vi "Initialize Attributes.vi"(8 "error in (no error)":errorcluster, 10 "Attribute Data":variant, 11 "CS++Scope":refnum<class "CS++Scope.lvclass">) -> (0 "error out":errorcluster, 2 "Found?":bool, 3 "CS++Scope out":refnum<class "CS++Scope.lvclass">)   [LabVIEW 2014, in "CS++Scope.lvlib" / "CS++Scope.lvclass"]
doc: "Initialize object attribute.\n\nUnique resources should be allocated elsewhere!"
uses:
  CS++Scope.lvclass
  PV-Enum.ctl
  PV-Enum-n.ctl
  CSPP_Core/Classes/CS++ProcessVariables/ProcessVariable/PV.lvclass
  CSPP_Core/Classes/CS++ProcessVariables/ProcessVariable/PV.lvclass/PV.ctl
  CSPP_Core/Actors/CS++BaseActor/CS++BaseActor.lvclass/CS++BaseActor.ctl
  CS++Scope.lvclass/CS++Scope.ctl
  CSPP_Core/Classes/CS++ProcessVariables/ProcessVariable/Write PV URL.vi
  CSPP_Core/Classes/CS++ProcessVariables/ProcessVariable/Write Type Descriptor.vi
  CSPP_Core/Actors/CS++DeviceActor/CS++DeviceActor.lvclass
  CSPP_Core/Classes/CS++BaseClasses/Factory/CS++Factory.lvclass
  CSPP_Core/Actors/CS++BaseActor/CS++BaseActor.lvclass
  CSPP_Core/Libraries/Utilities/CS++Utilities.lvlib
  CSPP_Core/Classes/CS++ProcessVariables/CS++ProcessVariables.lvlib
panel:
  in  "PV-Enum-n":T1
  in  "PV-Enum":T2
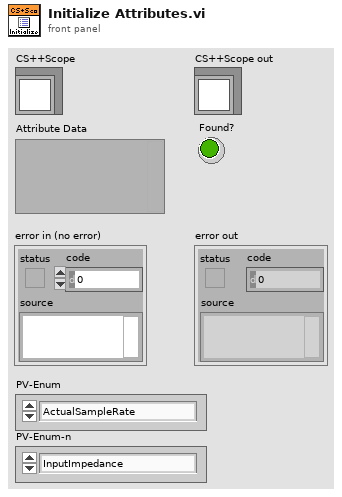
[diagram p1: front panel]
types:
  T1 = typedef "CS++Scope.lvlib/CS++Scope.lvclass/PV-Enum-n.ctl" = enum16{"InputImpedance", "MaxInputFrequency", "VerticalRange", "ProbeAttenuation", "VerticalOffset", "VerticalCoupling", "ChannelEnabled"}
  T2 = typedef "CS++Scope.lvlib/CS++Scope.lvclass/PV-Enum.ctl" = enum16{"ActualSampleRate", "TimePerRecord", "AcquisitionStartTime", "TriggerLevel", "GlitchWidth", "LowReference", "MidReference", "HighReference", "RuntLowThreshold", "RuntHighThreshold", "TriggerHoldoff", "WidthLowThreshold", "WidthHighThreshold", "AcquisitionStatus", "ActualRecordLength", "ActualSampleMode", "ACLineTriggerSlope", "MinRecordLength", "AcquisitionType", "TriggerSlope", "GlitchCondition", "GlitchPolarity", "InterpolationMethod", "NumberOfAverages", "NumberOfEnvelopes", "TriggerType", "TriggerCoupling", "TriggerModifier", "TVLineNumber", "TVEvent", "TVTriggerPolarity", "TVSignalFormat", "WidthCondition", "WidthPolarity", "MeasurementDone", "ContinousAcquisition", "TriggerSource", "Waveform", "ActualTimeIncrement"}
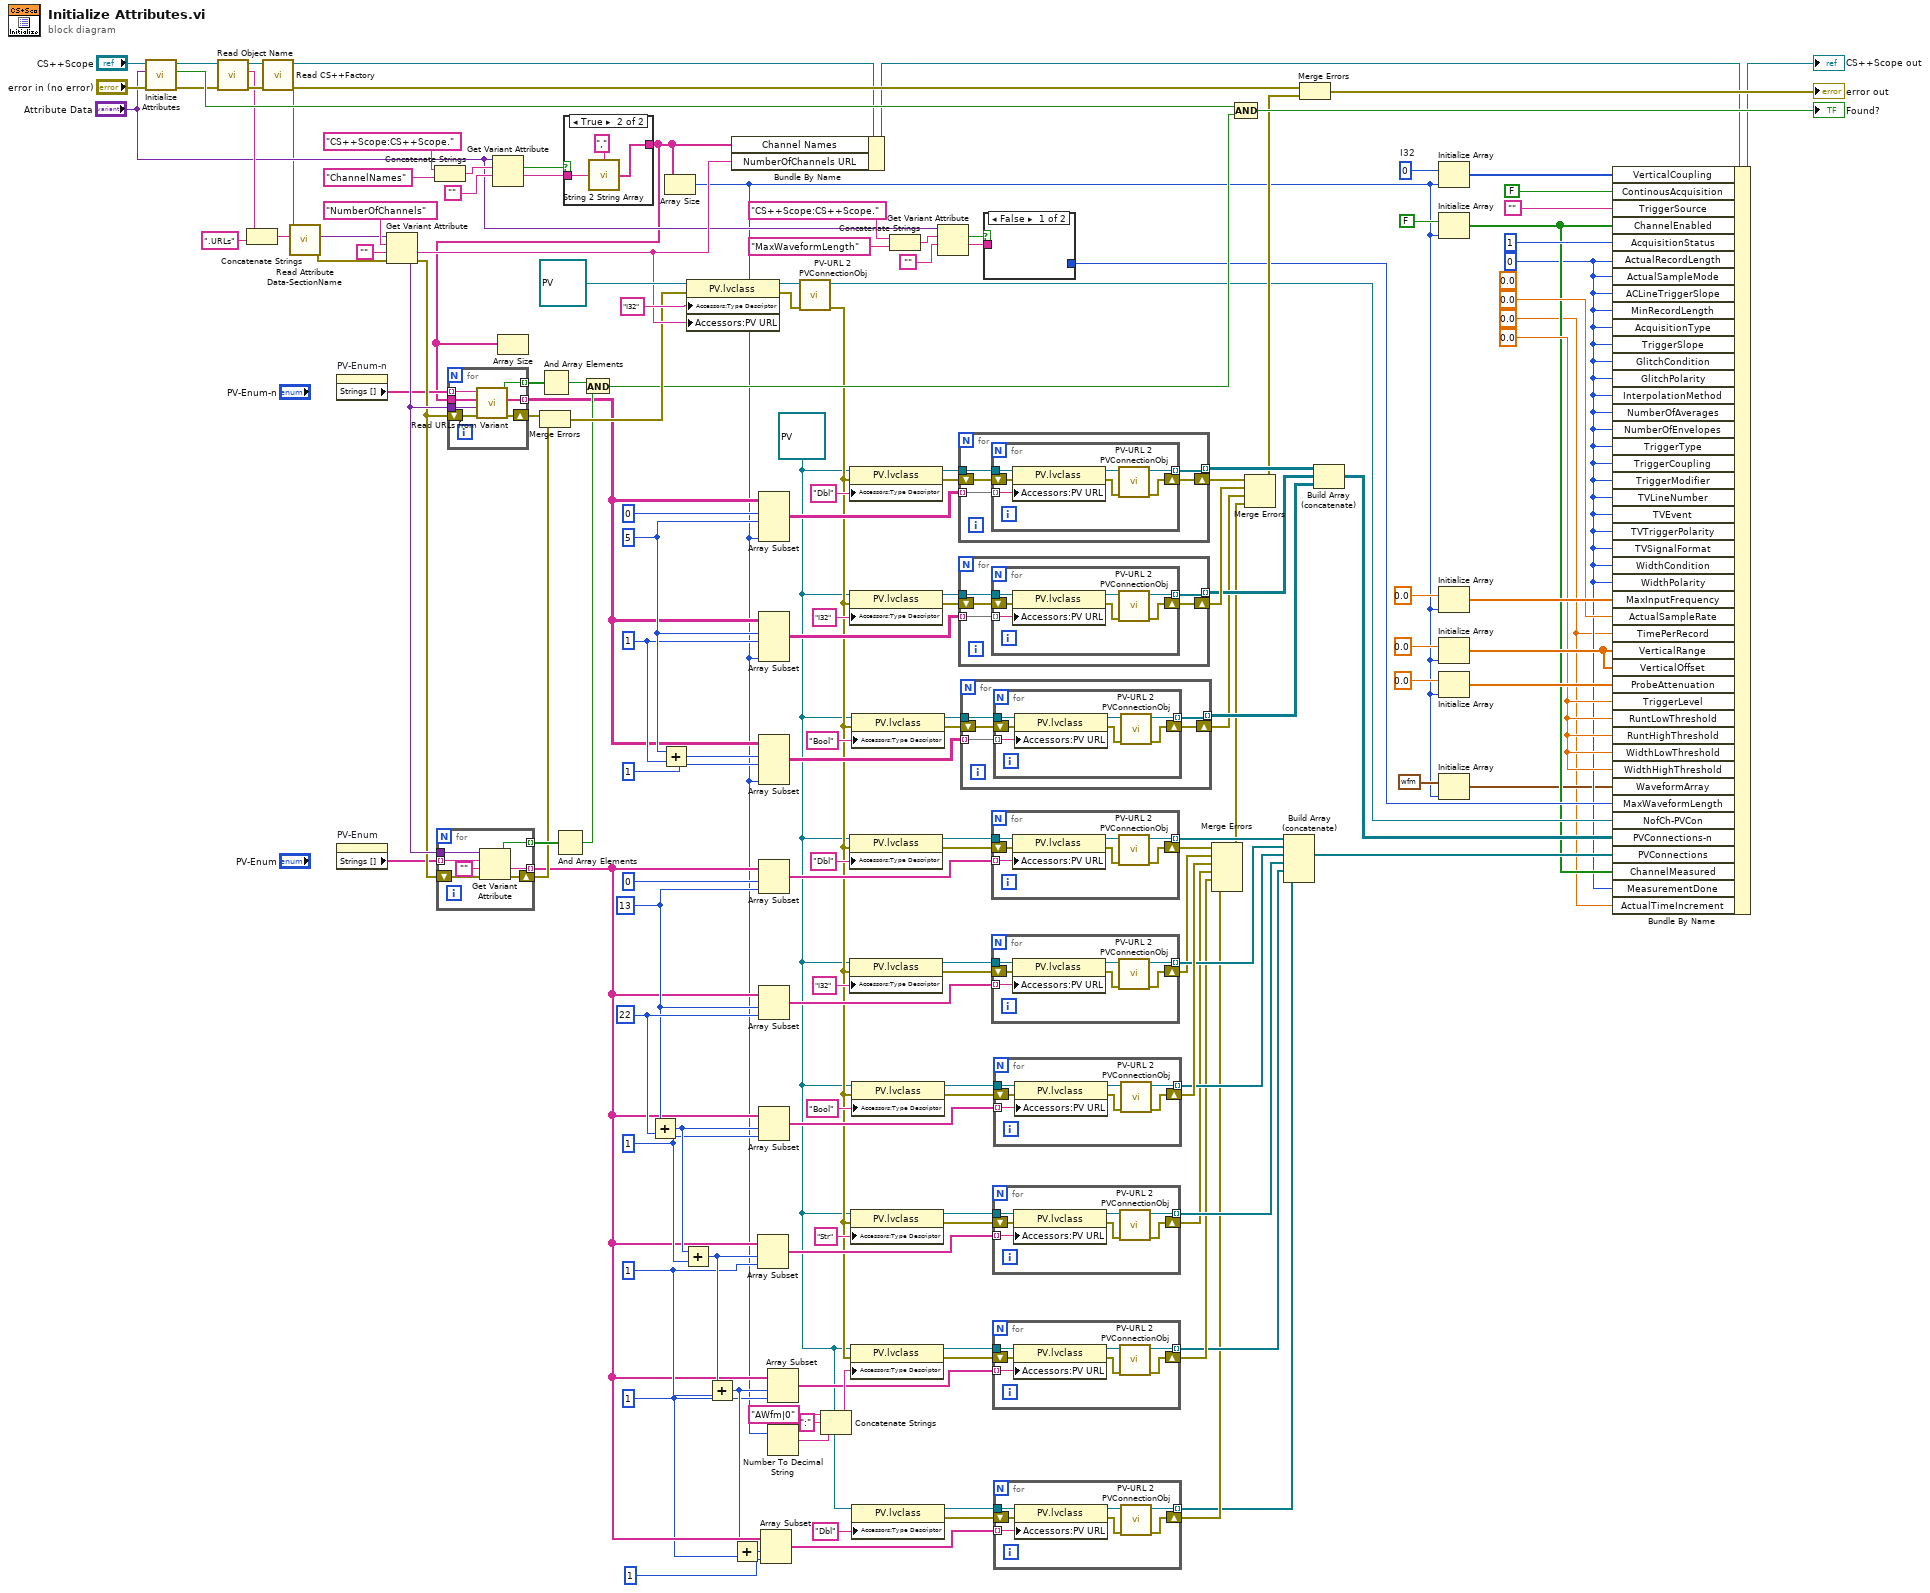
[diagram p0: block diagram]
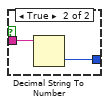
[diagram p2: hidden frame]
diagram:
  w7 = 1 ("length")
  w50 = dbl[unit] 0.0 ("modulation depth (0.00 %)")
  w19 = dbl[unit] 0.0 ("modulation depth (0.00 %)")
  w21 = 1 ("length")
  w58 = 1 ("length")
  w96 = 22 ("length")
  w95 = 13 ("length")
  w103 = 1 ("length")
  w104 = 5 ("length")
  w13 = refnum<class "PV.lvclass"> refnum ("CS++ProcessVariables.lvlib:PV.lvclass")
  (unwired) 0.0 ("modulation depth (0.00 %)")
  w35 = 0 ("I32")
  w136 = 0  # I32
  n1 = call-parent "Initialize Attributes.vi"("error in (no error)"="error in (no error)", "Attribute Data"="Attribute Data", "CS++DeviceActor in"="CS++Scope") -> ("error out"=w151:errorcluster, "Found?"=w154:bool, "CS++DeviceActor out"=w130:refnum<class "CS++Scope.lvclass">)  [unwired: 6 in]
  n2 = call "Read Object Name.vi"("error in (no error)"=w151, "CS++BaseActor in"=w130) -> ("error out"=w152:errorcluster, "Object Name"=w138:string, "CS++BaseActor out"=w153:refnum<class "CS++Scope.lvclass">)  [unwired: 7 in]
  n3 = Concatenate Strings(w138, ".URLs" ("string")) -> (w4:string)
  n4 = call "Read CS++Factory.vi"("error in (no error)"=w152, "CS++BaseActor in"=w153) -> ("error out"=w150:errorcluster, "CS++Factory"=w3:refnum<class "CS++Factory.lvclass">, "CS++BaseActor out"=w143:refnum<class "CS++Scope.lvclass">)  [unwired: 7 in]
  n5 = call-dynamic "Read Attribute Data-SectionName.vi"("Object Name"=w4, "CS++Factory in"=w3) -> ("error out"=w6:errorcluster, "Attribute Data"=w5:variant)  [unwired: 7 in, 1 out]
  n6 = property on="PV-Enum-n" class="Enum (strict)"() -> ("Strings []"=w66:string[])  [unwired: 2 in, 2 out]
  n7 = property on="PV-Enum" class="Enum (strict)"() -> ("Strings []"=w65:string[])  [unwired: 2 in, 2 out]
  n8 = Get Variant Attribute(Variant=w5, name="NumberOfChannels" ("string"), default value (empty Variant)="", error in=w6) -> (duplicate Variant=w101:variant, value=w125:string, error out=w100:errorcluster)  [unwired: 1 out]
  n9 = Concatenate Strings("CS++Scope:CS++Scope.", "ChannelNames" ("string")) -> (w145:string)
  n10 = for {
    tunnel: w65 -> [w159] mode=indexing
    tunnel: w101 -> [w160]
    shift-right: [w162] -> w73
    shift-left: w100 -> [w161]
    tunnel: [w158] -> w75 mode=indexing
    tunnel: [w156] -> w12 mode=indexing
    n11 = Get Variant Attribute(Variant=w160, name=w159, default value (empty Variant)="", error in=w161) -> (found=w158:bool, value=w156:string, error out=w162:errorcluster)  [unwired: 1 out]
  }
  n12 = Get Variant Attribute(Variant="Attribute Data", name=w145, default value (empty Variant)="") -> (found=w148:bool, value=w147:string)  [unwired: 1 in, 2 out]
  n13 = And Array Elements(Boolean array=w75) -> (logical AND=w71:bool)
  n14 = case shown="True" w148 {
    tunnel: w147 -> [_ w165]
    tunnel: [_ w164] -> w34
    frame False {
    }
    frame True {
      n15 = call "String 2 String Array.vi"("String"=w165, "Delimiter (\",\")"="," ("Delimiter (\",\")")) -> ("Substrings"=w164:string[])
    }
  }
  n16 = for {
    tunnel: w66 -> [w172] mode=indexing
    tunnel: [w171] -> w124 mode=indexing
    tunnel: w101 -> [w169]
    tunnel: w34 -> [w168]
    tunnel: [w167] -> w41 mode=indexing
    shift-right: [w170] -> w102
    shift-left: w100 -> [w166]
    n17 = call "Read URLs from Variant.vi"("Error In"=w166, "URL Section Data"=w169, "Channel Names"=w168, "URL Prefix"=w172) -> ("Error Out"=w170:errorcluster, "URLs"=w167:string[], "Found?"=w171:bool)  [unwired: 5 in]
  }
  n18 = Array Size(array=w34) -> ()  [unwired: 1 out]
  n19 = Merge Errors(w102, w73) -> (w74:errorcluster)
  n20 = And Array Elements(Boolean array=w124) -> (logical AND=w97:bool)
  n21 = And(x=w97, y=w71) -> (x .and. y?=w72:bool)
  n22 = Add(x=w95, y=w96) -> (x+y=w59:i32)
  n23 = Add(x=w104, y=w103) -> (x+y=w40:i32)
  n24 = Array Size(array=w34) -> (size(s)=w2:i32)
  n25 = Add(x=w59, y=w58) -> (x+y=w22:i32)
  n26 = property class="PV.lvclass"(reference=refnum<class "PV.lvclass"> refnum ("CS++ProcessVariables.lvlib:PV.lvclass"), error in=w74, "Accessors:Type Descriptor"="I32" ("Type Descriptor"), "Accessors:PV URL"=w125) -> (reference out=w126:refnum<class "PV.lvclass">, error out=w127:errorcluster)
  n27 = Add(x=w22, y=w21) -> (x+y=w8:i32)
  n28 = Bundle By Name(cluster=w143, "Channel Names"=w34, "NumberOfChannels URL"=w125) -> (w99:refnum<class "CS++Scope.lvclass">)
  n29 = Add(x=w8, y=w7) -> (x+y=w9:i32)
  n30 = Array Subset(array=w12, index=w22, length=w21) -> (w60:string[])
  n31 = Array Subset(array=w41, index (row)=0 ("index"), length (row)=w104, length (col)=w2) -> (w123:string[][])  [unwired: 1 in]
  n32 = Array Subset(array=w41, index (row)=w104, length (row)=w103, length (col)=w2) -> (w112:string[][])  [unwired: 1 in]
  n33 = Array Subset(array=w41, index (row)=w40, length (row)=1 ("length"), length (col)=w2) -> (w111:string[][])  [unwired: 1 in]
  n34 = Array Subset(array=w12, index=0, length=w95) -> (w76:string[])
  n35 = Array Subset(array=w12, index=w95, length=w96) -> (w87:string[])
  n36 = Array Subset(array=w12, index=w59, length=w58) -> (w88:string[])
  n37 = Array Subset(array=w12, index=w9, length=1) -> (w14:string[])
  n38 = Array Subset(array=w12, index=w8, length=w7) -> (w23:string[])
  n39 = Number To Decimal String(number=w2) -> (decimal integer string=w30:string)  [unwired: 1 in]
  n40 = call "PV-URL 2 PVConnectionObj.vi"("Error In"=w127, "PV"=w126) -> ("Error Out"=w24:errorcluster, "PVConnection"=w49:refnum<class "PVConnection.lvclass">)  [unwired: 7 in, 1 out]
  n41 = Concatenate Strings("AWfm|0" ("Type Descriptor"), ":" ("string"), w30) -> (w29:string)
  n42 = property class="PV.lvclass"(reference=w13, error in=w24, "Accessors:Type Descriptor"="Dbl" ("Type Descriptor")) -> (reference out=w121:refnum<class "PV.lvclass">, error out=w120:errorcluster)
  n43 = property class="PV.lvclass"(reference=w13, error in=w24, "Accessors:Type Descriptor"="I32" ("Type Descriptor")) -> (reference out=w116:refnum<class "PV.lvclass">, error out=w117:errorcluster)
  n44 = property class="PV.lvclass"(reference=w13, error in=w24, "Accessors:Type Descriptor"="Dbl" ("Type Descriptor")) -> (reference out=w78:refnum<class "PV.lvclass">, error out=w79:errorcluster)
  n45 = property class="PV.lvclass"(reference=w13, error in=w24, "Accessors:Type Descriptor"="I32" ("Type Descriptor")) -> (reference out=w83:refnum<class "PV.lvclass">, error out=w82:errorcluster)
  n46 = property class="PV.lvclass"(reference=w13, error in=w24, "Accessors:Type Descriptor"="Str" ("Type Descriptor")) -> (reference out=w62:refnum<class "PV.lvclass">, error out=w63:errorcluster)
  n47 = property class="PV.lvclass"(reference=w13, error in=w24, "Accessors:Type Descriptor"=w29) -> (reference out=w26:refnum<class "PV.lvclass">, error out=w25:errorcluster)
  n48 = property class="PV.lvclass"(reference=w13, error in=w24, "Accessors:Type Descriptor"="Bool" ("Type Descriptor")) -> (reference out=w109:refnum<class "PV.lvclass">, error out=w108:errorcluster)
  n49 = property class="PV.lvclass"(reference=w13, error in=w24, "Accessors:Type Descriptor"="Bool" ("Type Descriptor")) -> (reference out=w90:refnum<class "PV.lvclass">, error out=w91:errorcluster)
  n50 = property class="PV.lvclass"(reference=w13, "Accessors:Type Descriptor"="Dbl" ("Type Descriptor")) -> (reference out=w16:refnum<class "PV.lvclass">, error out=w17:errorcluster)  [unwired: 1 in]
  n51 = Concatenate Strings("CS++Scope:CS++Scope.", "MaxWaveformLength" ("string")) -> (w46:string)
  n52 = Get Variant Attribute(Variant="Attribute Data", name=w46, default value (empty Variant)="") -> (found=w43:bool, value=w42:string)  [unwired: 1 in, 2 out]
  n53 = for {
    tunnel: w121 -> [w177]
    tunnel: w123 -> [w176] mode=indexing
    tunnel: [w175] -> w118 mode=indexing
    shift-right: [w174] -> w119
    shift-left: w120 -> [w173]
    n54 = for {
      tunnel: w177 -> [w183]
      tunnel: w176 -> [w182] mode=indexing
      tunnel: [w181] -> w175 mode=indexing
      shift-right: [w180] -> w174
      shift-left: w173 -> [w178]
      n55 = property class="PV.lvclass"(reference=w183, error in=w178, "Accessors:PV URL"=w182) -> (reference out=w184:refnum<class "PV.lvclass">, error out=w179:errorcluster)
      n56 = call "PV-URL 2 PVConnectionObj.vi"("Error In"=w179, "PV"=w184) -> ("Error Out"=w180:errorcluster, "PVConnection"=w181:refnum<class "PVConnection.lvclass">)  [unwired: 7 in, 1 out]
    }
  }
  n57 = for {
    tunnel: w116 -> [w189]
    tunnel: w112 -> [w188] mode=indexing
    tunnel: [w187] -> w113 mode=indexing
    shift-right: [w186] -> w114
    shift-left: w117 -> [w185]
    n58 = for {
      tunnel: w189 -> [w195]
      tunnel: w188 -> [w194] mode=indexing
      tunnel: [w193] -> w187 mode=indexing
      shift-right: [w192] -> w186
      shift-left: w185 -> [w190]
      n59 = property class="PV.lvclass"(reference=w195, error in=w190, "Accessors:PV URL"=w194) -> (reference out=w196:refnum<class "PV.lvclass">, error out=w191:errorcluster)
      n60 = call "PV-URL 2 PVConnectionObj.vi"("Error In"=w191, "PV"=w196) -> ("Error Out"=w192:errorcluster, "PVConnection"=w193:refnum<class "PVConnection.lvclass">)  [unwired: 7 in, 1 out]
    }
  }
  n61 = for {
    tunnel: w109 -> [w201]
    tunnel: w111 -> [w200] mode=indexing
    tunnel: [w199] -> w107 mode=indexing
    shift-right: [w198] -> w106
    shift-left: w108 -> [w197]
    n62 = for {
      tunnel: w201 -> [w207]
      tunnel: w200 -> [w206] mode=indexing
      tunnel: [w205] -> w199 mode=indexing
      shift-right: [w204] -> w198
      shift-left: w197 -> [w202]
      n63 = property class="PV.lvclass"(reference=w207, error in=w202, "Accessors:PV URL"=w206) -> (reference out=w208:refnum<class "PV.lvclass">, error out=w203:errorcluster)
      n64 = call "PV-URL 2 PVConnectionObj.vi"("Error In"=w203, "PV"=w208) -> ("Error Out"=w204:errorcluster, "PVConnection"=w205:refnum<class "PVConnection.lvclass">)  [unwired: 7 in, 1 out]
    }
  }
  n65 = case shown="False" w43 {
    tunnel: w42 -> [_ w210]
    tunnel: [_ w209] -> w38
    frame False {
    }
    frame True {
      n66 = Decimal String To Number(string=w210) -> (number=w209:i32)  [unwired: 2 in, 1 out]
    }
  }
  n67 = for {
    tunnel: w78 -> [w216]
    tunnel: w76 -> [w215] mode=indexing
    tunnel: [w214] -> w81 mode=indexing
    shift-right: [w213] -> w80
    shift-left: w79 -> [w211]
    n68 = property class="PV.lvclass"(reference=w216, error in=w211, "Accessors:PV URL"=w215) -> (reference out=w217:refnum<class "PV.lvclass">, error out=w212:errorcluster)
    n69 = call "PV-URL 2 PVConnectionObj.vi"("Error In"=w212, "PV"=w217) -> ("Error Out"=w213:errorcluster, "PVConnection"=w214:refnum<class "PVConnection.lvclass">)  [unwired: 7 in, 1 out]
  }
  n70 = for {
    tunnel: w83 -> [w223]
    tunnel: w87 -> [w222] mode=indexing
    tunnel: [w221] -> w86 mode=indexing
    shift-right: [w220] -> w85
    shift-left: w82 -> [w218]
    n71 = property class="PV.lvclass"(reference=w223, error in=w218, "Accessors:PV URL"=w222) -> (reference out=w224:refnum<class "PV.lvclass">, error out=w219:errorcluster)
    n72 = call "PV-URL 2 PVConnectionObj.vi"("Error In"=w219, "PV"=w224) -> ("Error Out"=w220:errorcluster, "PVConnection"=w221:refnum<class "PVConnection.lvclass">)  [unwired: 7 in, 1 out]
  }
  n73 = for {
    tunnel: w62 -> [w230]
    tunnel: w60 -> [w229] mode=indexing
    tunnel: [w228] -> w57 mode=indexing
    shift-right: [w227] -> w56
    shift-left: w63 -> [w225]
    n74 = property class="PV.lvclass"(reference=w230, error in=w225, "Accessors:PV URL"=w229) -> (reference out=w231:refnum<class "PV.lvclass">, error out=w226:errorcluster)
    n75 = call "PV-URL 2 PVConnectionObj.vi"("Error In"=w226, "PV"=w231) -> ("Error Out"=w227:errorcluster, "PVConnection"=w228:refnum<class "PVConnection.lvclass">)  [unwired: 7 in, 1 out]
  }
  n76 = for {
    tunnel: w26 -> [w237]
    tunnel: w23 -> [w236] mode=indexing
    tunnel: [w235] -> w27 mode=indexing
    shift-right: [w234] -> w28
    shift-left: w25 -> [w232]
    n77 = property class="PV.lvclass"(reference=w237, error in=w232, "Accessors:PV URL"=w236) -> (reference out=w238:refnum<class "PV.lvclass">, error out=w233:errorcluster)
    n78 = call "PV-URL 2 PVConnectionObj.vi"("Error In"=w233, "PV"=w238) -> ("Error Out"=w234:errorcluster, "PVConnection"=w235:refnum<class "PVConnection.lvclass">)  [unwired: 7 in, 1 out]
  }
  n79 = for {
    tunnel: w90 -> [w244]
    tunnel: w88 -> [w243] mode=indexing
    tunnel: [w242] -> w92 mode=indexing
    shift-right: [w241] -> w93
    shift-left: w91 -> [w239]
    n80 = property class="PV.lvclass"(reference=w244, error in=w239, "Accessors:PV URL"=w243) -> (reference out=w245:refnum<class "PV.lvclass">, error out=w240:errorcluster)
    n81 = call "PV-URL 2 PVConnectionObj.vi"("Error In"=w240, "PV"=w245) -> ("Error Out"=w241:errorcluster, "PVConnection"=w242:refnum<class "PVConnection.lvclass">)  [unwired: 7 in, 1 out]
  }
  n82 = for {
    tunnel: w16 -> [w251]
    tunnel: w14 -> [w250] mode=indexing
    tunnel: [w249] -> w10 mode=indexing
    shift-right: [w248] -> w11
    shift-left: w17 -> [w246]
    n83 = property class="PV.lvclass"(reference=w251, error in=w246, "Accessors:PV URL"=w250) -> (reference out=w252:refnum<class "PV.lvclass">, error out=w247:errorcluster)
    n84 = call "PV-URL 2 PVConnectionObj.vi"("Error In"=w247, "PV"=w252) -> ("Error Out"=w248:errorcluster, "PVConnection"=w249:refnum<class "PVConnection.lvclass">)  [unwired: 7 in, 1 out]
  }
  n85 = Merge Errors(w80, w85, w93, w56, w28, w11) -> (w20:errorcluster)
  n86 = Compound Arithmetic op=AND(w154, w72) -> (→"Found?":bool)
  n87 = Merge Errors(w119, w114, w106, w20) -> (w98:errorcluster)
  n88 = Build Array (concatenate)(w81, w86, w92, w57, w27, w10) -> (w69:refnum<class "PVConnection.lvclass">[])
  n89 = Merge Errors(w150, w98) -> (→"error out":errorcluster)
  n90 = Build Array (concatenate)(w118, w113, w107) -> (w70:refnum<class "PVConnection.lvclass">[][])
  n91 = Initialize Array(w136, w2) -> (w131:i32[])
  n92 = Initialize Array(FALSE, w2) -> (w36:bool[])
  n93 = Initialize Array(dbl[unit] 0.0 ("modulation depth (0.00 %)"), w2) -> (w55:dbl[unit][])
  n94 = Initialize Array(dbl[unit] 0.0 ("modulation depth (0.00 %)"), w2) -> (w132:dbl[unit][])
  n95 = Initialize Array(0.0 ("modulation depth (0.00 %)"), w2) -> (w51:dbl[])
  n96 = Initialize Array(waveform(dbl) {"t0"=timestamp(0 s since 1904-01-01), "dt"=1.0, "Y"=[]} ("WaveformArray"), w2) -> (w32:waveform(dbl)[])
  n97 = Bundle By Name(cluster=w99, "VerticalCoupling"=w131, "ContinousAcquisition"=FALSE ("Sample Clock Output Enabled (Disabled)"), "TriggerSource"="" ("output state (Constant Voltage)"), "ChannelEnabled"=w36, "AcquisitionStatus"=1 ("I32"), "ActualRecordLength"=w35, "ActualSampleMode"=w35, "ACLineTriggerSlope"=w35, "MinRecordLength"=w35, "AcquisitionType"=w35, "TriggerSlope"=w35, "GlitchCondition"=w35, "GlitchPolarity"=w35, "InterpolationMethod"=w35, "NumberOfAverages"=w35, "NumberOfEnvelopes"=w35, "TriggerType"=w35, "TriggerCoupling"=w35, "TriggerModifier"=w35, "TVLineNumber"=w35, "TVEvent"=w35, "TVTriggerPolarity"=w35, "TVSignalFormat"=w35, "WidthCondition"=w35, "WidthPolarity"=w35, "MaxInputFrequency"=w55, "ActualSampleRate"=dbl[unit] 0.0 ("modulation depth (0.00 %)"), "TimePerRecord"=w19, "VerticalRange"=w132, "VerticalOffset"=w132, "ProbeAttenuation"=w51, "TriggerLevel"=w50, "RuntLowThreshold"=w50, "RuntHighThreshold"=w50, "WidthLowThreshold"=w50, "WidthHighThreshold"=w50, "WaveformArray"=w32, "MaxWaveformLength"=w38, "NofCh-PVCon"=w49, "PVConnections-n"=w70, "PVConnections"=w69, "ChannelMeasured"=w36, "MeasurementDone"=w35, "ActualTimeIncrement"=w19) -> (→"CS++Scope out":refnum<class "CS++Scope.lvclass">)
